vi "new dp.vi"   [LabVIEW 2013]
uses:
  StateMachineStates 1.ctl
types:
  T1 = typedef "StateMachineStates 1.ctl" = enum16{"Initialize", "Main", "Stop"}
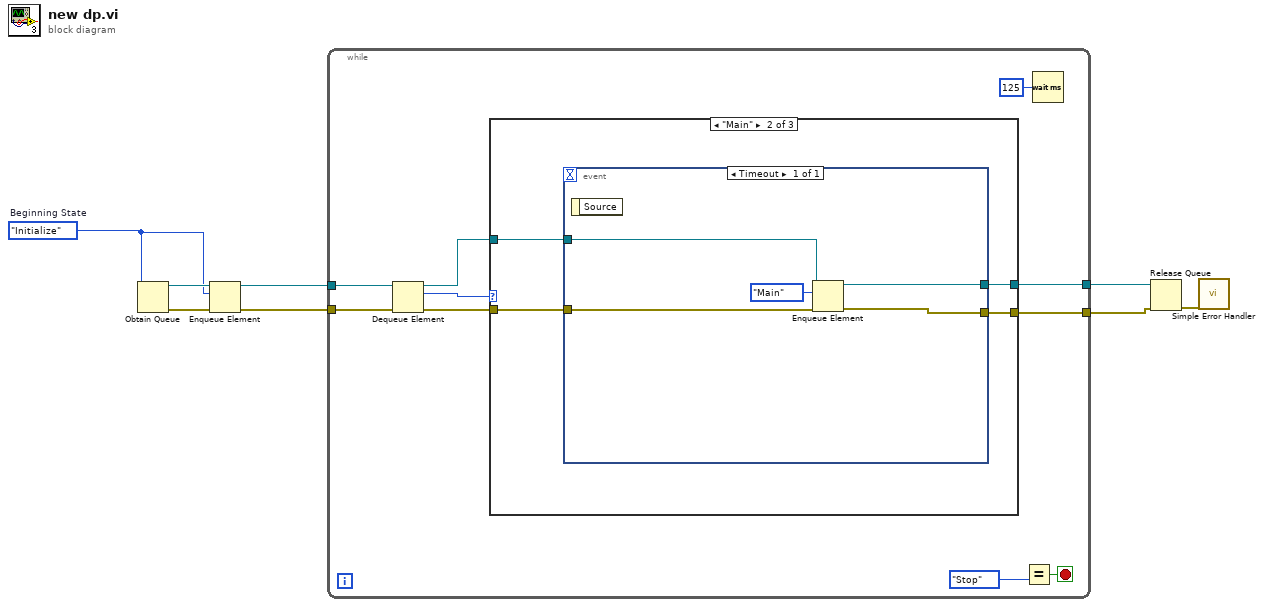
[diagram p0: block diagram]
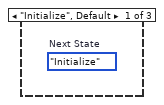
[diagram p2: hidden frame]
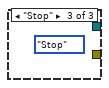
[diagram p3: hidden frame]
diagram:
  w6 = StateMachineStates_1."Initialize"  # Beginning State
  n1 = Obtain Queue(element data type=w6) -> (queue out=w8:refnum<queue>, error out=w7:errorcluster)  [unwired: 4 in, 1 out]
  n2 = Enqueue Element(queue=w8, element=w6, error in (no error)=w7) -> (queue out=w4:refnum<queue>, error out=w5:errorcluster)  [unwired: 1 in, 1 out]
  n3 = while {
    tunnel: w5 -> [w15]
    tunnel: w4 -> [w14]
    tunnel: [w10] -> w3
    tunnel: [w9] -> w2
    stop <- w18 stop-if-true
    n4 = Dequeue Element(queue=w14, error in (no error)=w15) -> (queue out=w12:refnum<queue>, element=w13:T1, error out=w11:errorcluster)  [unwired: 1 in, 1 out]
    n5 = case shown="\"Main\"" w13 {
      tunnel: w12 -> [_ w22 _]
      tunnel: w11 -> [_ w21 _]
      tunnel: [_ w20 _] -> w10
      tunnel: [_ w19 _] -> w9
      frame "Initialize", Default {
        (unwired) StateMachineStates_1."Initialize"  # Next State
      }
      frame "Main" {
        n6 = event shown="[0] Timeout" {
          selector: _ -> [_]
          dyn-events: _ -> [_]
          timeout: _ -> [_]
          tunnel: w22 -> [w27]
          tunnel: w21 -> [w26]
          tunnel: [w25] -> w20
          tunnel: [w24] -> w19
          event Timeout {
            n7 = event-data() -> ()  [unwired: 1 in, 1 out]
            n8 = Enqueue Element(queue=w27, element=StateMachineStates_1."Main", error in (no error)=w26) -> (queue out=w24:refnum<queue>, error out=w25:errorcluster)  [unwired: 1 in, 1 out]
          }
        }
      }
      frame "Stop" {
        (unwired) StateMachineStates_1."Stop" ("Next State")
      }
    }
    n9 = Equal?(y=StateMachineStates_1."Stop" ("States")) -> (x = y?=w18:bool)  [unwired: 1 in]
    n10 = Wait (ms)(milliseconds to wait=u32 125) -> ()  [unwired: 1 out]
  }
  n11 = Release Queue(queue=w2, error in (no error)=w3) -> (error out=w1:errorcluster)  [unwired: 1 in, 2 out]
  n12 = call <vilib>:"Simple Error Handler.vi"("error in (no error)"=w1) -> ()  [unwired: 4 in, 5 out]
